vi "flat top measure.vi"(9 "Integration time":dbl, 11 "rare or stable":bool) -> (3 "Measurement":dbl)   [LabVIEW 2016, in "flat top.lvlib"]
uses:
  flat top.lvlib
  <vilib>/Analysis/baseanly.llb/Mean (DBL).vi
  sub-VIs/sub-VIs.lvlib
  <vilib>/Analysis/NI_AALBase.lvlib
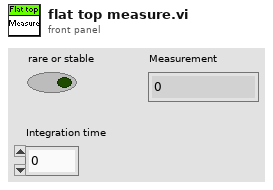
[diagram p1: front panel]
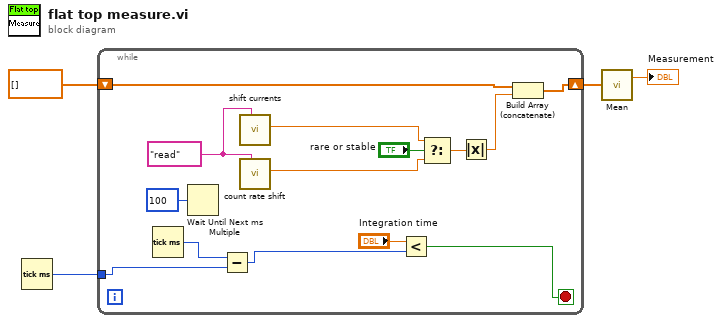
[diagram p0: block diagram]
diagram:
  n1 = Tick Count (ms)() -> (millisecond timer value=w3:u32)
  n2 = while {
    shift-right: [w12] -> w2
    shift-left: dbl[] [] -> [w11]
    tunnel: w3 -> [w8]
    stop <- w6 stop-if-true
    w16 = "read" ("Combo Box")
    n3 = Tick Count (ms)() -> (millisecond timer value=w9:u32)
    n4 = Wait Until Next ms Multiple(millisecond multiple=u32 100) -> ()  [unwired: 1 out]
    n5 = Subtract(x=w9, y=w8) -> (x-y=w7:u32)
    n6 = call "shift currents.vi"("Combo Box"=w16) -> ("current out"=w14:dbl)  [unwired: 10 in]
    n7 = call "count rate shift.vi"("read or write"=w16) -> ("count rate out"=w17:dbl)  [unwired: 10 in]
    n8 = Less?(x="Integration time", y=w7) -> (x < y?=w6:bool)
    n9 = Select(t=w14, s="rare or stable", f=w17) -> (s? t:f=w15:dbl)
    n10 = Absolute Value(x=w15) -> (abs(x)=w10:dbl)
    n11 = Build Array (concatenate)(w11, w10) -> (w12:dbl[])
  }
  n12 = call-poly <vilib>:"Mean.vi"("X"=w2) -> ("mean"=→"Measurement":dbl)  [unwired: 1 out]
